vi "DCPowerVCC.vi"() -> ()   [LabVIEW 2020]
uses:
  FunctionVi/Queue/Control/QueueState.ctl
  <userlib>/FTLDCPower/MPD.lvlib
panel:
  out "Measure VOLTage":dbl format="%#.3gV"
  out "Measure Power":dbl format="%#.3gW"
  out "Measure Current":dbl format="%#.3gA"
  in  "Time Target (s)":dbl=5.0 caption="Time Target" format="%#.3gs"
  in  "Step Voltage":dbl=0.1 format="%#.3gV"
  in  "Current":dbl format="%#.3gV"
  in  "Voltage":dbl format="%#.3gV"
  in  "On/Off":bool
  in  "Config":bool
  # "Measurement"
  # "Params Set"
  # "Output"
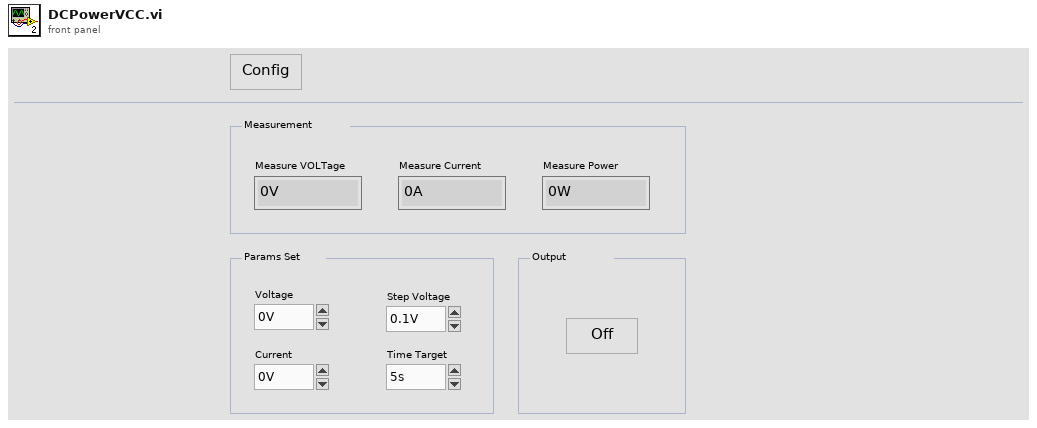
[diagram p1: front panel]
types:
  T1 = typedef "QueueState.ctl" = enum16{"", "Create", "In", "Out", "Empty", "Close"}
  T2 = cluster{"Baud Rate":u32, "Parity":u16, "Data Bits":u16, "Stop Bits":u16, "Flow Control":u16}
  T3 = enum16{"VOLTage", "DEFault", "MINimum", "MAXimum"}
  T4 = enum16{"current", "DEFault", "MINimum", "MAXimum"}
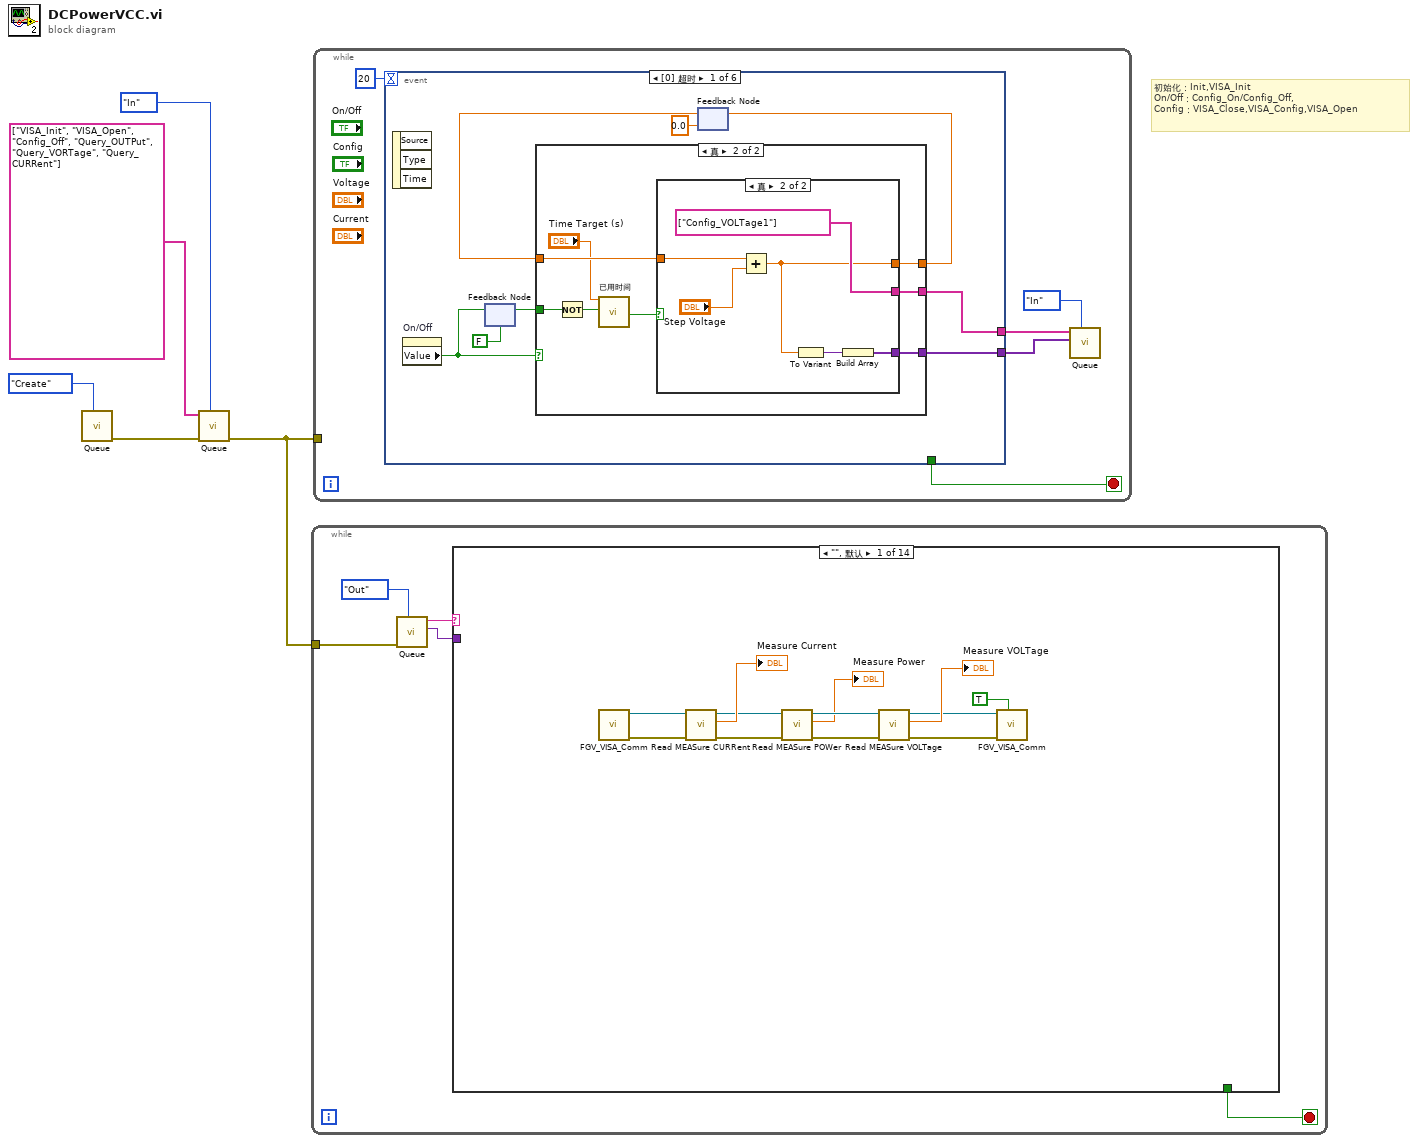
[diagram p0: block diagram]
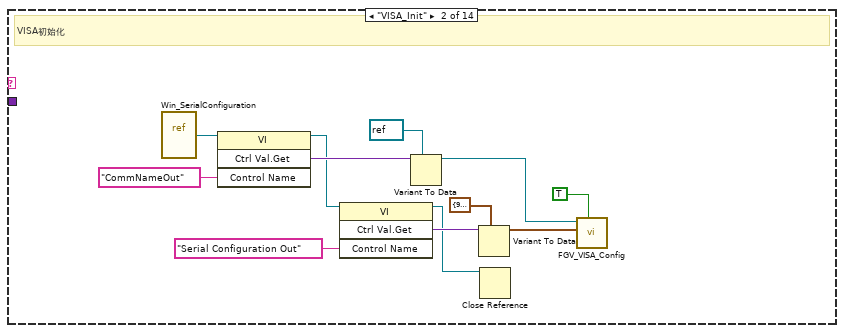
[diagram p2: hidden frame]
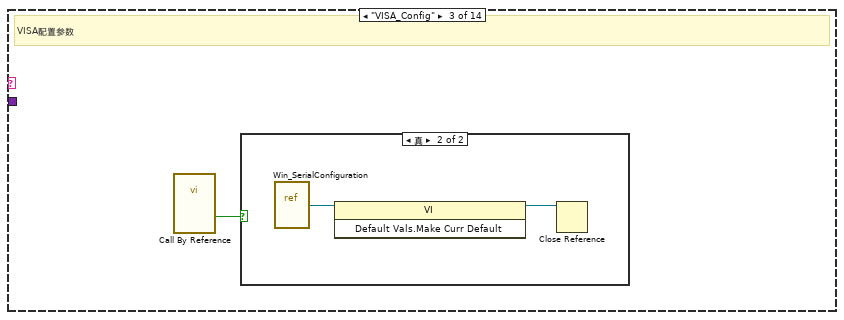
[diagram p3: hidden frame]
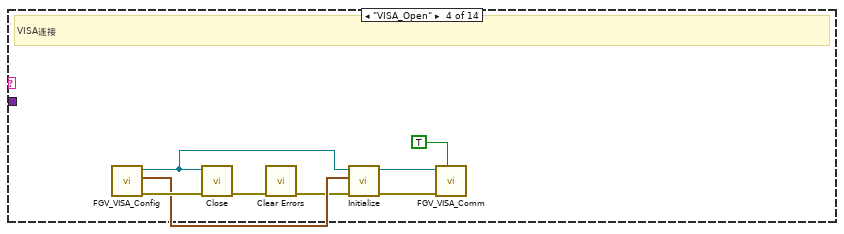
[diagram p5: hidden frame]
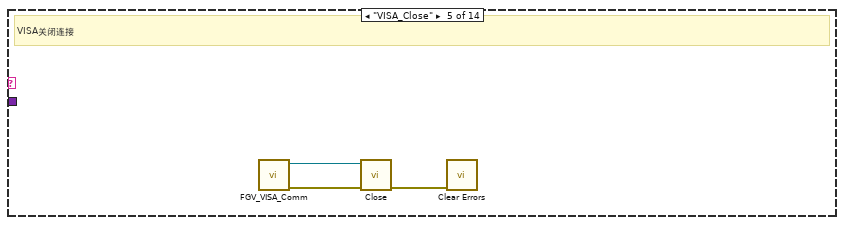
[diagram p6: hidden frame]
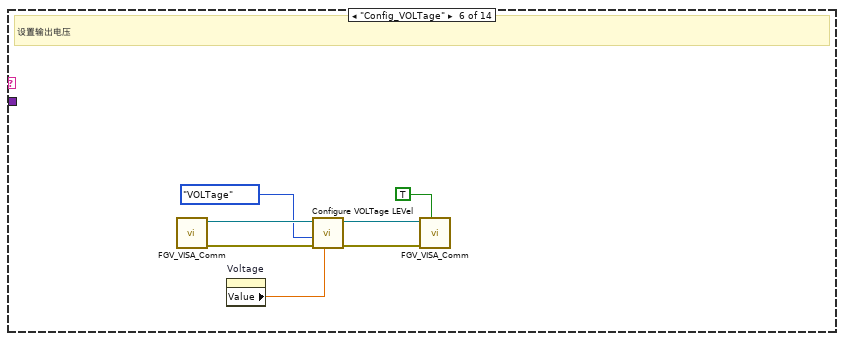
[diagram p7: hidden frame]
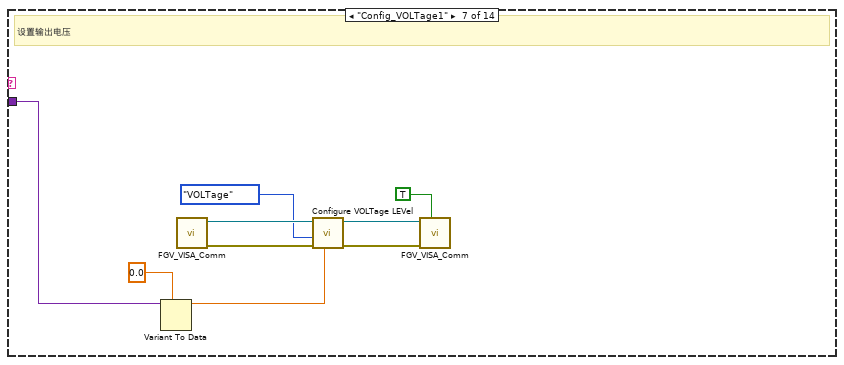
[diagram p8: hidden frame]
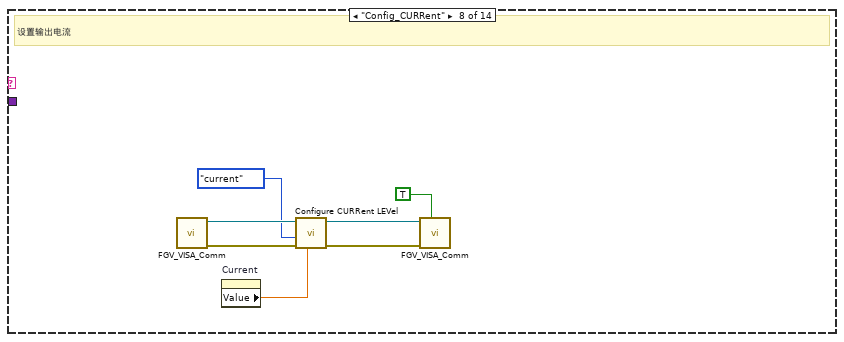
[diagram p9: hidden frame]
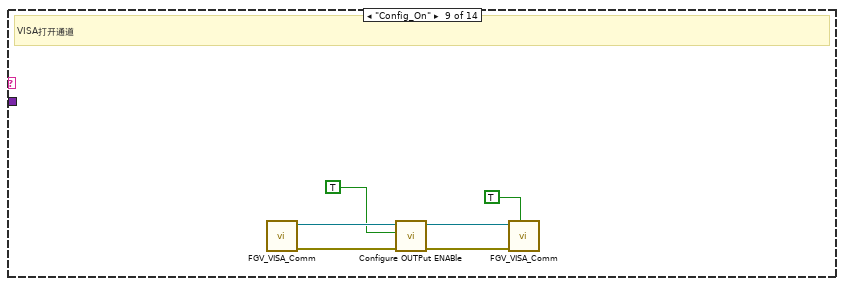
[diagram p10: hidden frame]
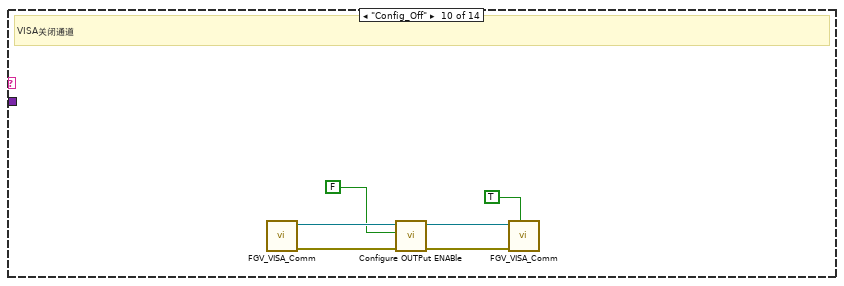
[diagram p11: hidden frame]
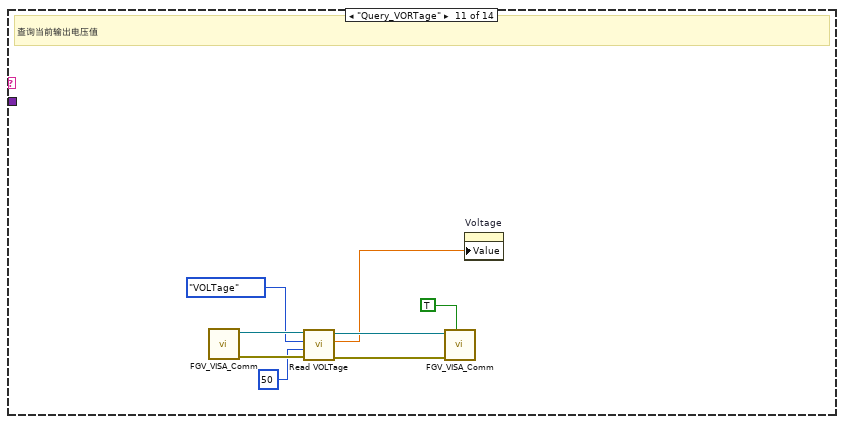
[diagram p12: hidden frame]
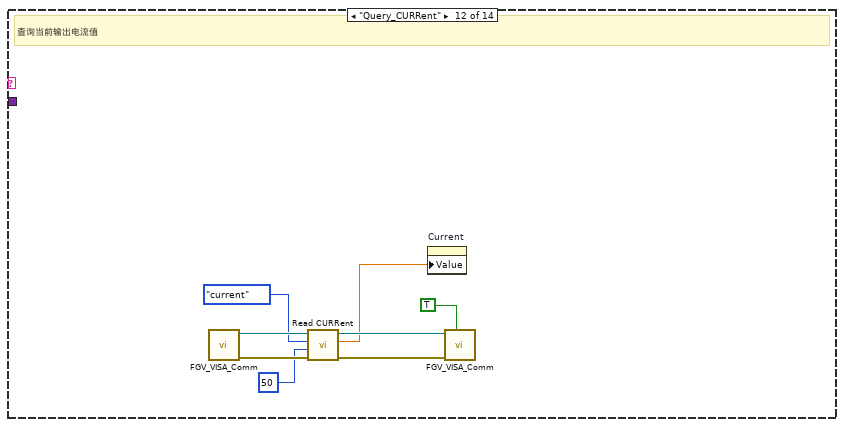
[diagram p13: hidden frame]
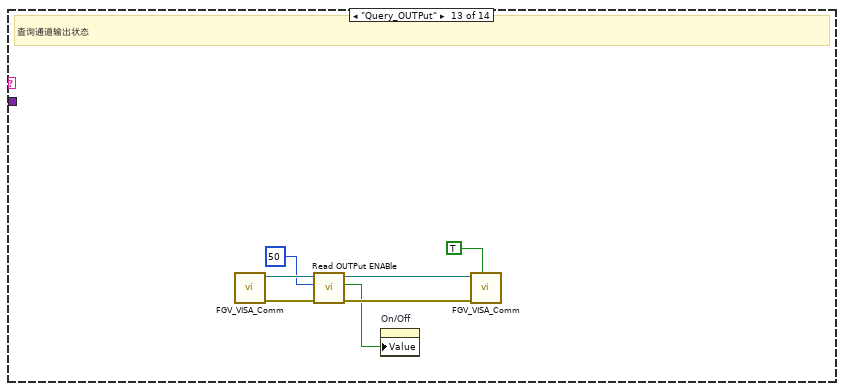
[diagram p14: hidden frame]
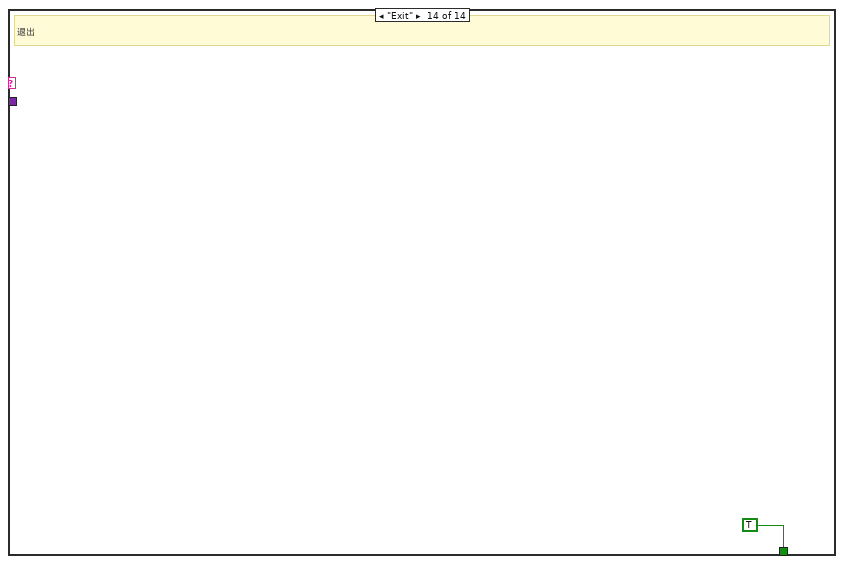
[diagram p15: hidden frame]
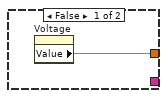
[diagram p16: hidden frame]
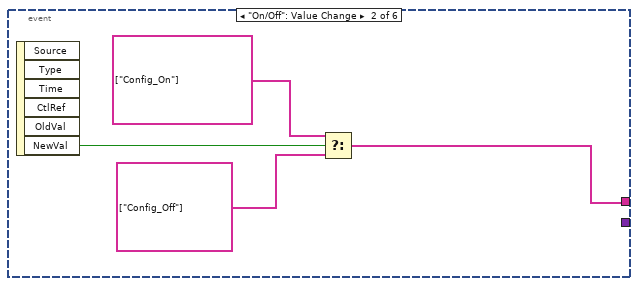
[diagram p18: hidden frame]
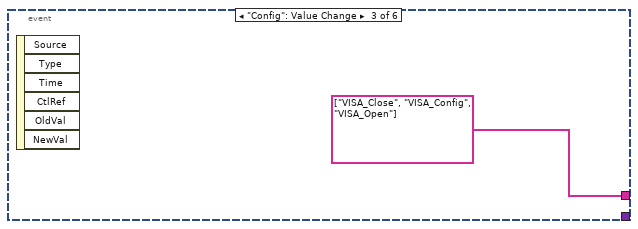
[diagram p19: hidden frame]
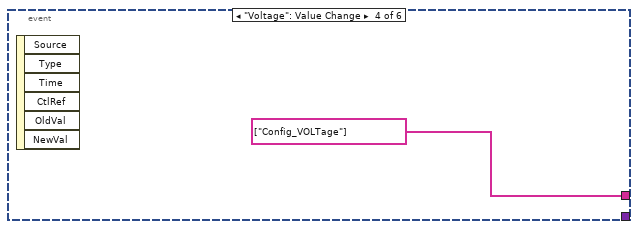
[diagram p20: hidden frame]
diagram:
  # "初始化：Init,VISA_Init\nOn/Off：Config_On/Config_Off,\nConfig：VISA_Close,VISA_Config,VISA_Open"
  n1 = call "Queue.vi"("State"=QueueState."Create") -> ("error out"=w4:errorcluster)  [unwired: 8 in, 2 out]
  n2 = call "Queue.vi"("State"=QueueState."In", "error in"=w4, "Instruct"=string[] ["VISA_Init", "VISA_Open", "Config_Off", "Query_OUTPut", "Query_VORTage", "Query_CURRent"]) -> ("error out"=w3:errorcluster)  [unwired: 6 in, 2 out]
  n3 = while {
    tunnel: w3 -> [w10]
    stop <- w7 stop-if-true
    n4 = call "Queue.vi"("State"=QueueState."Out", "error in"=w10) -> ("Data Out"=w6:variant, "Instruct Out"=w8:string)  [unwired: 7 in, 1 out]
    n5 = case shown="\"\", 默认" w8 {
      tunnel: [_ _ _ _ _ _ _ _ _ _ _ _ _ TRUE] -> w7
      tunnel: w6 -> [_ _ _ _ _ _ w58 _ _ _ _ _ _ _]
      frame "", Default {
        n6 = call "FGV_VISA_Comm.vi"() -> ("error out"=w22:errorcluster, "VISA resource name out"=w14:refnum<visa-resource-name>)  [unwired: 10 in]
        n7 = call <userlib>:"Read MEASure CURRent.vi"("error in (no error)"=w22, "VISA resource name"=w14) -> ("error out"=w21:errorcluster, "Measure Current"=→"Measure Current":dbl, "VISA resource name out"=w15:refnum<visa-resource-name>)  [unwired: 7 in]
        n8 = call <userlib>:"Read MEASure POWer.vi"("error in (no error)"=w21, "VISA resource name"=w15) -> ("error out"=w19:errorcluster, "Measure Power"=→"Measure Power":dbl, "VISA resource name out"=w20:refnum<visa-resource-name>)  [unwired: 7 in]
        n9 = call <userlib>:"Read MEASure VOLTage.vi"("error in (no error)"=w19, "VISA resource name"=w20) -> ("error out"=w12:errorcluster, "Measure VOLTage"=→"Measure VOLTage":dbl, "VISA resource name out"=w13:refnum<visa-resource-name>)  [unwired: 7 in]
        n10 = call "FGV_VISA_Comm.vi"("Write?"=TRUE, "error in"=w12, "VISA resource name"=w13) -> ()  [unwired: 7 in, 2 out]
      }
      frame "VISA_Init" {
        # "VISA初始化"
        n11 = vi-ref "Win_SerialConfiguration.vi"() -> (w34:refnum<vi>)
        n12 = invoke class="VI" method="Ctrl Val.Get"(reference=w34, "Control Name"="CommNameOut" ("控件名")) -> (reference out=w30:refnum<vi>, "Get Control Value Variant"=w32:variant)  [unwired: 2 in, 2 out]
        n13 = invoke class="VI" method="Ctrl Val.Get"(reference=w30, "Control Name"="Serial Configuration Out" ("控件名")) -> (reference out=w23:refnum<vi>, "Get Control Value Variant"=w28:variant)  [unwired: 2 in, 2 out]
        n14 = Variant To Data(type=refnum<visa-resource-name> refnum ("VISA资源名称"), Variant=w32) -> (data=w26:refnum<visa-resource-name>)  [unwired: 1 in, 1 out]
        n15 = Variant To Data(type=T2 {"Baud Rate"=9600, "Parity"=0, "Data Bits"=8, "Stop Bits"=10, "Flow Control"=0} ("Serial Configuration"), Variant=w28) -> (data=w25:T2)  [unwired: 1 in, 1 out]
        n16 = Close Reference(reference=w23) -> ()  [unwired: 1 in, 1 out]
        n17 = call "FGV_VISA_Config.vi"("Write?"=TRUE, "Serial Configuration"=w25, "CommName"=w26) -> ()  [unwired: 6 in, 3 out]
      }
      frame "VISA_Config" {
        # "VISA配置参数"
        n18 = call-by-ref "?"() -> ("Yes out"=w35:bool)  [unwired: 10 in, 5 out]
        n19 = case shown="真" w35 {
          frame False {
          }
          frame True {
            n20 = vi-ref "Win_SerialConfiguration.vi"() -> (w37:refnum<vi>)
            n21 = invoke class="VI" method="Default Vals.Make Curr Default"(reference=w37) -> (reference out=w36:refnum<vi>)  [unwired: 2 in, 2 out]
            n22 = Close Reference(reference=w36) -> ()  [unwired: 1 in, 1 out]
          }
        }
      }
      frame "VISA_Open" {
        # "VISA连接"
        n23 = call "FGV_VISA_Config.vi"() -> ("error out"=w42:errorcluster, "Serial Configuration Out"=w40:T2, "CommNameOut"=w41:refnum<visa-resource-name>)  [unwired: 9 in]
        n24 = call <userlib>:"Close.vi"("error in (no error)"=w42, "VISA resource name"=w41) -> ("error out"=w39:errorcluster)  [unwired: 9 in]
        n25 = call <vilib>:"Clear Errors.vi"("error in (no error)"=w39) -> ("error out"=w38:errorcluster)  [unwired: 5 in, 1 out]
        n26 = call <userlib>:"Initialize.vi"("VISA resource name"=w41, "Serial Configuration"=w40, "error in (no error)"=w38) -> ("VISA resource name out"=w45:refnum<visa-resource-name>, "error out"=w44:errorcluster)  [unwired: 6 in]
        n27 = call "FGV_VISA_Comm.vi"("Write?"=TRUE, "error in"=w44, "VISA resource name"=w45) -> ()  [unwired: 7 in, 2 out]
      }
      frame "VISA_Close" {
        # "VISA关闭连接"
        n28 = call "FGV_VISA_Comm.vi"() -> ("error out"=w47:errorcluster, "VISA resource name out"=w48:refnum<visa-resource-name>)  [unwired: 10 in]
        n29 = call <userlib>:"Close.vi"("error in (no error)"=w47, "VISA resource name"=w48) -> ("error out"=w46:errorcluster)  [unwired: 9 in]
        n30 = call <vilib>:"Clear Errors.vi"("error in (no error)"=w46) -> ()  [unwired: 5 in, 2 out]
      }
      frame "Config_VOLTage" {
        # "设置输出电压"
        n31 = call "FGV_VISA_Comm.vi"() -> ("error out"=w52:errorcluster, "VISA resource name out"=w54:refnum<visa-resource-name>)  [unwired: 10 in]
        n32 = property on="Voltage" class="DigNum (严格)"() -> ("Value"=w49:dbl)  [unwired: 2 in, 2 out]
        n33 = call <userlib>:"Configure VOLTage LEVel.vi"("VOLTage  Value(V)"=w49, "error in (no error)"=w52, "VOLTage Tab"=T3."VOLTage", "VISA resource name"=w54) -> ("error out"=w51:errorcluster, "VISA resource name out"=w53:refnum<visa-resource-name>)  [unwired: 6 in]
        n34 = call "FGV_VISA_Comm.vi"("Write?"=TRUE, "error in"=w51, "VISA resource name"=w53) -> ()  [unwired: 7 in, 2 out]
      }
      frame "Config_VOLTage1" {
        # "设置输出电压"
        n35 = Variant To Data(type=0.0 ("x+y"), Variant=w58) -> (data=w56:dbl)  [unwired: 1 in, 1 out]
        n36 = call "FGV_VISA_Comm.vi"() -> ("error out"=w61:errorcluster, "VISA resource name out"=w63:refnum<visa-resource-name>)  [unwired: 10 in]
        n37 = call <userlib>:"Configure VOLTage LEVel.vi"("VOLTage  Value(V)"=w56, "error in (no error)"=w61, "VOLTage Tab"=T3."VOLTage", "VISA resource name"=w63) -> ("error out"=w60:errorcluster, "VISA resource name out"=w62:refnum<visa-resource-name>)  [unwired: 6 in]
        n38 = call "FGV_VISA_Comm.vi"("Write?"=TRUE, "error in"=w60, "VISA resource name"=w62) -> ()  [unwired: 7 in, 2 out]
      }
      frame "Config_CURRent" {
        # "设置输出电流"
        n39 = call "FGV_VISA_Comm.vi"() -> ("error out"=w67:errorcluster, "VISA resource name out"=w68:refnum<visa-resource-name>)  [unwired: 10 in]
        n40 = property on="Current" class="DigNum (严格)"() -> ("Value"=w65:dbl)  [unwired: 2 in, 2 out]
        n41 = call <userlib>:"Configure CURRent LEVel.vi"("Current  Value(A)"=w65, "error in (no error)"=w67, "Current Tab"=T4."current", "VISA resource name"=w68) -> ("error out"=w69:errorcluster, "VISA resource name out"=w70:refnum<visa-resource-name>)  [unwired: 6 in]
        n42 = call "FGV_VISA_Comm.vi"("Write?"=TRUE, "error in"=w69, "VISA resource name"=w70) -> ()  [unwired: 7 in, 2 out]
      }
      frame "Config_On" {
        # "VISA打开通道"
        n43 = call "FGV_VISA_Comm.vi"() -> ("error out"=w76:errorcluster, "VISA resource name out"=w77:refnum<visa-resource-name>)  [unwired: 10 in]
        n44 = call <userlib>:"Configure OUTPut ENABle.vi"("error in (no error)"=w76, "Enable OUTPut (T: Enable)"=TRUE, "VISA resource name"=w77) -> ("error out"=w72:errorcluster, "VISA resource name out"=w74:refnum<visa-resource-name>)  [unwired: 7 in]
        n45 = call "FGV_VISA_Comm.vi"("Write?"=TRUE, "error in"=w72, "VISA resource name"=w74) -> ()  [unwired: 7 in, 2 out]
      }
      frame "Config_Off" {
        # "VISA关闭通道"
        n46 = call "FGV_VISA_Comm.vi"() -> ("error out"=w82:errorcluster, "VISA resource name out"=w83:refnum<visa-resource-name>)  [unwired: 10 in]
        n47 = call <userlib>:"Configure OUTPut ENABle.vi"("error in (no error)"=w82, "Enable OUTPut (T: Enable)"=FALSE, "VISA resource name"=w83) -> ("error out"=w78:errorcluster, "VISA resource name out"=w80:refnum<visa-resource-name>)  [unwired: 7 in]
        n48 = call "FGV_VISA_Comm.vi"("Write?"=TRUE, "error in"=w78, "VISA resource name"=w80) -> ()  [unwired: 7 in, 2 out]
      }
      frame "Query_VORTage" {
        # "查询当前输出电压值"
        n49 = call "FGV_VISA_Comm.vi"() -> ("error out"=w89:errorcluster, "VISA resource name out"=w90:refnum<visa-resource-name>)  [unwired: 10 in]
        n50 = call <userlib>:"Read VOLTage.vi"("error in (no error)"=w89, "等待时间（毫秒）"=u32 50, "VOLTage Tab"=T3."VOLTage", "VISA resource name"=w90) -> ("error out"=w86:errorcluster, "VOLTage  Value"=w85:dbl, "VISA resource name out"=w87:refnum<visa-resource-name>)  [unwired: 5 in]
        n51 = call "FGV_VISA_Comm.vi"("Write?"=TRUE, "error in"=w86, "VISA resource name"=w87) -> ()  [unwired: 7 in, 2 out]
        n52 = property on="Voltage" class="DigNum (严格)"("Value"=w85) -> ()  [unwired: 2 in, 2 out]
      }
      frame "Query_CURRent" {
        # "查询当前输出电流值"
        n53 = call "FGV_VISA_Comm.vi"() -> ("error out"=w96:errorcluster, "VISA resource name out"=w98:refnum<visa-resource-name>)  [unwired: 10 in]
        n54 = call <userlib>:"Read CURRent.vi"("error in (no error)"=w96, "等待时间（毫秒）"=u32 50, "Current Tab"=T4."current", "VISA resource name"=w98) -> ("error out"=w95:errorcluster, "Current"=w93:dbl, "VISA resource name out"=w97:refnum<visa-resource-name>)  [unwired: 5 in]
        n55 = property on="Current" class="DigNum (严格)"("Value"=w93) -> ()  [unwired: 2 in, 2 out]
        n56 = call "FGV_VISA_Comm.vi"("Write?"=TRUE, "error in"=w95, "VISA resource name"=w97) -> ()  [unwired: 7 in, 2 out]
      }
      frame "Query_OUTPut" {
        # "查询通道输出状态"
        n57 = call "FGV_VISA_Comm.vi"() -> ("error out"=w103:errorcluster, "VISA resource name out"=w105:refnum<visa-resource-name>)  [unwired: 10 in]
        n58 = call <userlib>:"Read OUTPut ENABle.vi"("error in (no error)"=w103, "等待时间（毫秒）"=u32 50, "VISA resource name"=w105) -> ("error out"=w102:errorcluster, "OUTPut Status"=w101:bool, "VISA resource name out"=w104:refnum<visa-resource-name>)  [unwired: 6 in]
        n59 = property on="On/Off" class="Bool (严格)"("Value"=w101) -> ()  [unwired: 2 in, 2 out]
        n60 = call "FGV_VISA_Comm.vi"("Write?"=TRUE, "error in"=w102, "VISA resource name"=w104) -> ()  [unwired: 7 in, 2 out]
      }
      frame "Exit" {
        # "退出"
      }
    }
  }
  n61 = while {
    tunnel: w3 -> [_]
    stop <- w108 stop-if-true
    n62 = event shown="[0] 超时" {
      selector: _ -> [_ _ _ _ _ _]
      dyn-events: _ -> [_ _ _ _ _ _]
      timeout: 20 -> [_ _ _ _ _ _]
      tunnel: [w120 w137 string[] ["VISA_Close", "VISA_Config", "VISA_Open"] ("Instruct") string[] ["Config_VOLTage"] ("Instruct") string[] ["Config_CURRent"] ("Instruct") string[] ["Config_Off", "VISA_Close", "Exit"] ("Instruct")] -> w110
      tunnel: [w117 _ _ _ _ variant[] [] ("Data")] -> w109
      tunnel: [_ _ _ _ _ TRUE] -> w108
      event Timeout {
        n63 = event-data() -> ()  [unwired: 1 in, 3 out]
        n64 = property on="On/Off" class="Bool (严格)"() -> ("Value"=w115:bool)  [unwired: 2 in, 2 out]
        n65 = feedback-in #1(w115) -> ()
        n66 = feedback #1(FALSE ("Value")) -> (w113:bool)
        n67 = feedback #2(0.0) -> (w118:dbl)
        n68 = case shown="真" w115 {
          tunnel: [_ w128] -> w120
          tunnel: [w121 w127] -> w119
          tunnel: w118 -> [_ w125]
          tunnel: [_ w126] -> w117
          tunnel: w113 -> [_ w124]
          frame False {
            n69 = property on="Voltage" class="DigNum (严格)"() -> ("Value"=w121:dbl)  [unwired: 2 in, 2 out]
          }
          frame True {
            n70 = Not(x=w124) -> (.not. x?=w123:bool)
            n71 = call "已用时间"("Time Target (s)"="Time Target (s)", "Reset"=w123) -> ("Time has Elapsed"=w129:bool)  [unwired: 10 in, 7 out]
            n72 = case shown="真" w129 {
              tunnel: [_ string[] ["Config_VOLTage1"] ("Instruct")] -> w128
              tunnel: [w130 w133] -> w127
              tunnel: w125 -> [w130 w134]
              tunnel: [_ w131] -> w126
              frame False {
              }
              frame True {
                n73 = Add(x=w134, y="Step Voltage") -> (x+y=w133:dbl)
                n74 = To Variant(anything=w133) -> (Variant=w132:variant)
                n75 = Build Array(w132) -> (w131:variant[])
              }
            }
          }
        }
        n76 = feedback-in #2(w119) -> ()
      }
      event "On/Off": Value Change {
        n77 = event-data() -> ("NewVal"=w140:bool)  [unwired: 1 in, 5 out]
        n78 = Select(t=string[] ["Config_On"] ("Instruct"), s=w140, f=string[] ["Config_Off"] ("Instruct")) -> (s? t:f=w137:string[])
      }
      event "Config": Value Change {
        n79 = event-data() -> ()  [unwired: 1 in, 6 out]
      }
      event "Voltage": Value Change {
        n80 = event-data() -> ()  [unwired: 1 in, 6 out]
      }
      event "Current": Value Change {
        n81 = event-data() -> ()  [unwired: 1 in, 6 out]
      }
      event Panel Close? {
        n82 = event-data() -> ()  [unwired: 1 in, 4 out]
        n83 = event-data("Discard?"=TRUE ("放弃？")) -> ()  [unwired: 1 in, 1 out]
      }
    }
    n84 = call "Queue.vi"("State"=QueueState."In", "Data"=w109, "Instruct"=w110) -> ()  [unwired: 6 in, 3 out]
  }
